vi "Run1Ton.vi"() -> ()   [LabVIEW 2014]
doc: "Use this template to build a producer/consumer design pattern with events to produce queue items. Use this design pattern instead of the User Interface Event Handler pattern for user interfaces when you want to execute code asynchronously in response to an event without slowing the user interface responsiveness."
uses:
  <vilib>/addons/h5labview2/base/hid_t.ctl
  DatasetNames.ctl
  Program Files (x86)/CAEN/Comm/labview/CAENComm.lvlib
panel:
  in  "Delay":u32=1
  out "# elements in queue":i32
  out "Acquiring?":bool
  out "Wfm Plot 2":dbl[][](graph)
  out "# bad reads":i32
  out "Wfm Plot":dbl[][](graph)
  out "Scaler Data":u32[](array[numeric])
  out "Acquisition\nErrors":errorcluster
  in  "Clear Acquisition Errors":bool
  in  "QDC threshold":u16=1
  in  "Start Acquisition":bool
  out "# Events Written":i32
  in  "# Events to\nRecord":i32
  out "Analysis\nErrors":errorcluster
  in  "Calibrate Verniers":bool
  in  "Stop Acquisition":bool
  in  "Configure Output":bool
  in  "Calibrate Pedestals":bool
  in  "stop":bool
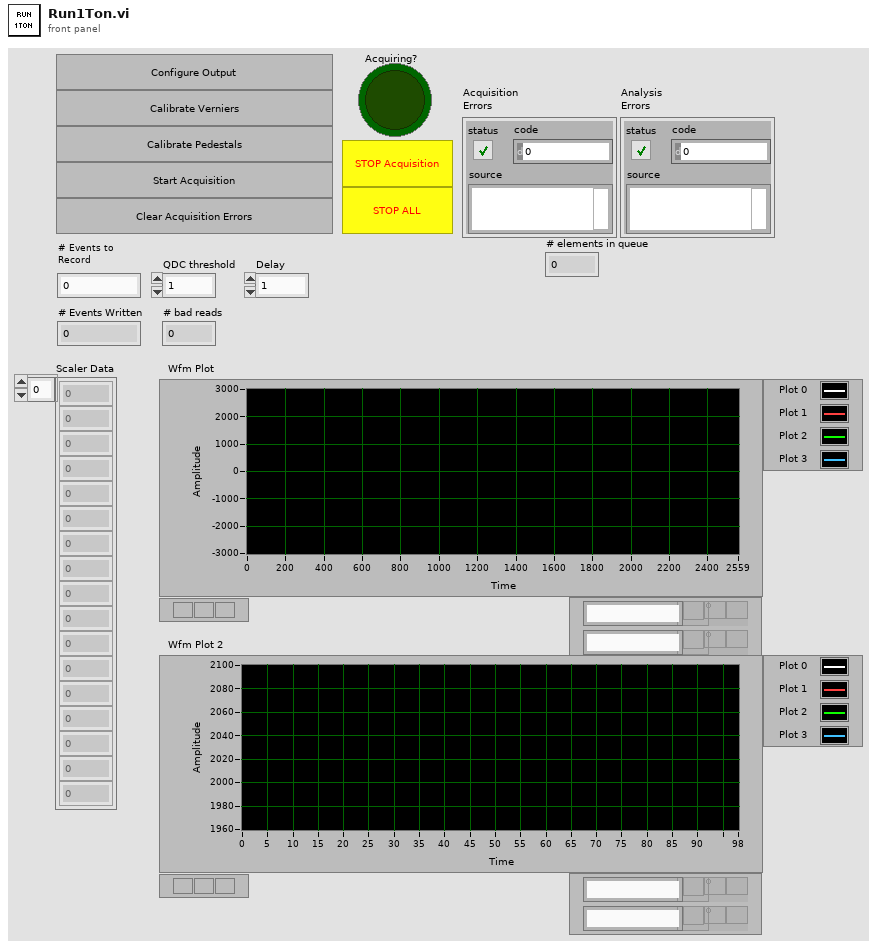
[diagram p1: front panel]
types:
  T1 = typedef "hid_t.ctl" = i32
  T2 = cluster{"State":enum16{"Startup", "Initialise", "Event OK", "Discard Event", "Exit", "Close"}, "Data":variant}
  T3 = typedef "DatasetNames.ctl" = enum16{"TDC", "Scaler", "QDC_1", "QDC_2", "Digitizer_1", "Digitizer_2"}
  T4 = cluster{"TDC Data":u32[], "Scaler Data":u32[], "QDC 1 Data":u32[], "QDC 2 Data":u32[], "Digitizer 1 TRIG_REC":u32, "Digitizer 1 Waveforms":u32[], "Digitizer 2 TRIG_REC":u32, "Digitizer 2 Waveforms":u32[]}
  T5 = enum16{"Startup", "Initialise", "Event OK", "Discard Event", "Exit", "Close"}
  T6 = enum16{"Configure", "Initialise", "Run", "Close"}
  T7 = cluster{"TDC":u32, "Scaler":u32, "QDC 1":u32, "QDC 2":u32, "Digitizer 1":u32, "Digitizer 2":u32}
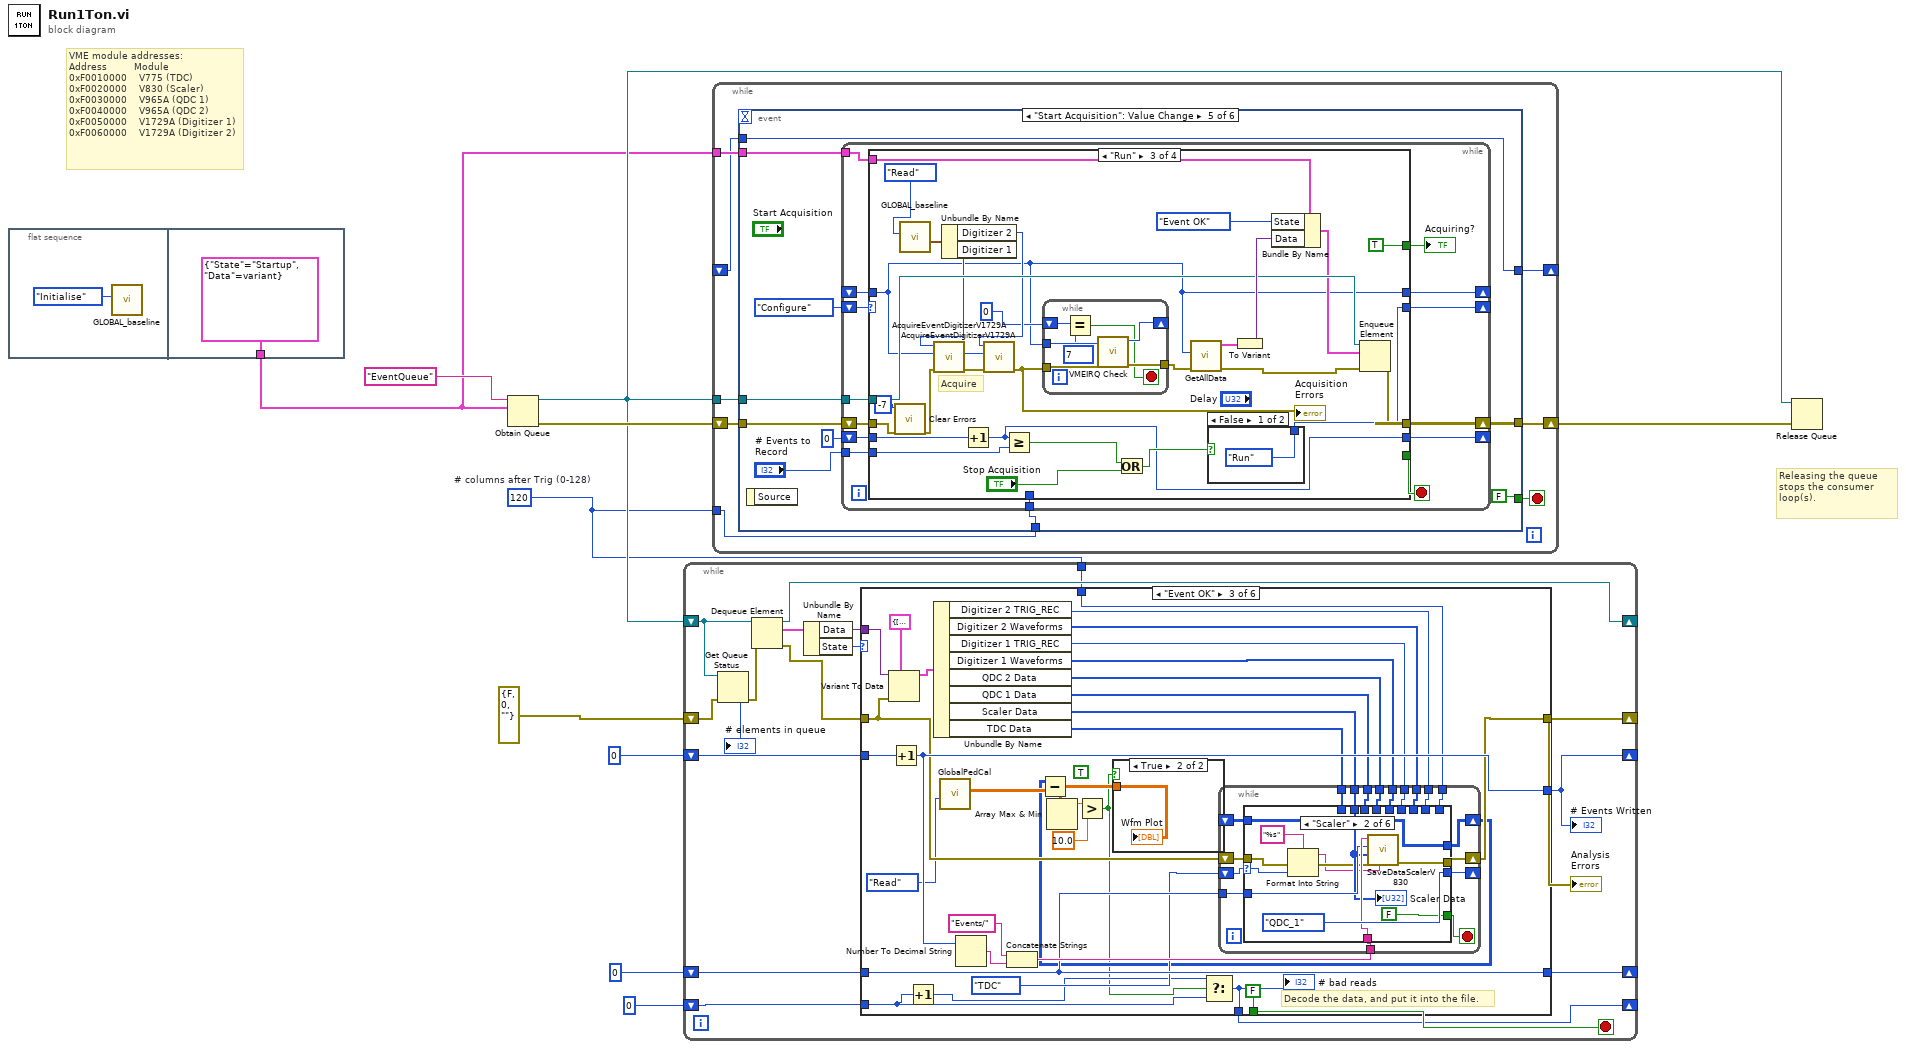
[diagram p0: block diagram]
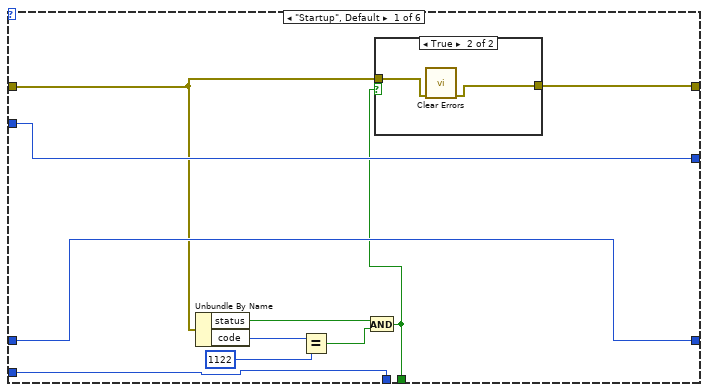
[diagram p2: hidden frame]
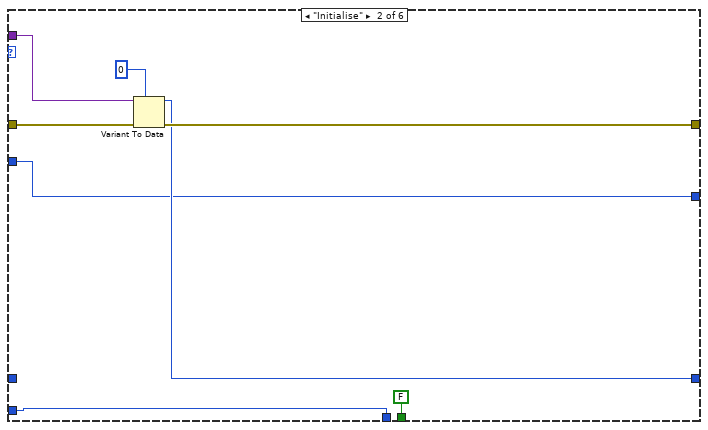
[diagram p4: hidden frame]
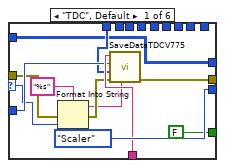
[diagram p6: hidden frame]
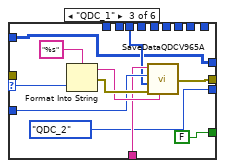
[diagram p7: hidden frame]
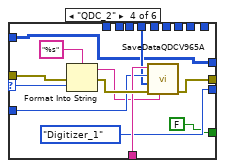
[diagram p8: hidden frame]
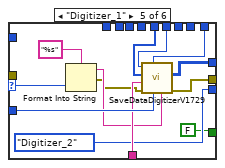
[diagram p9: hidden frame]
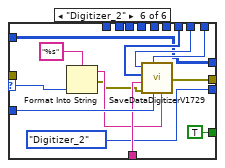
[diagram p10: hidden frame]
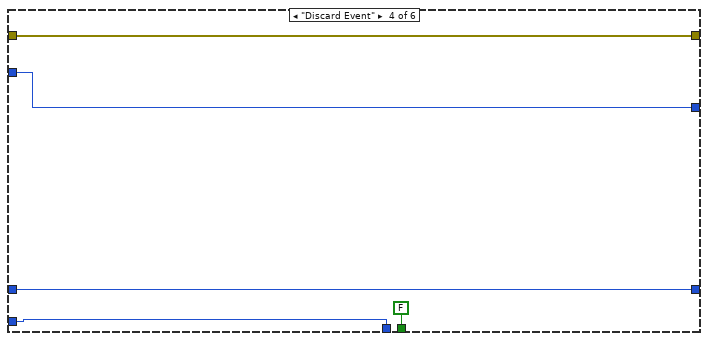
[diagram p11: hidden frame]
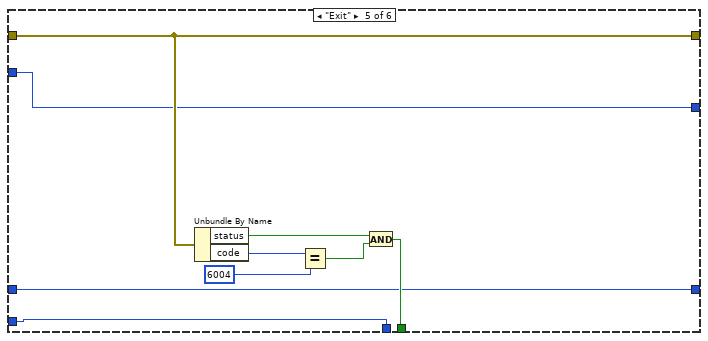
[diagram p12: hidden frame]
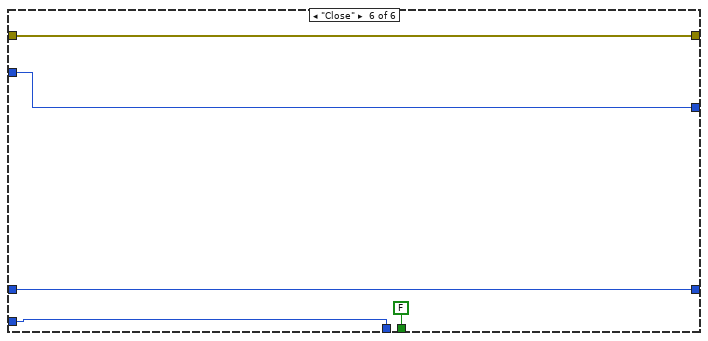
[diagram p13: hidden frame]
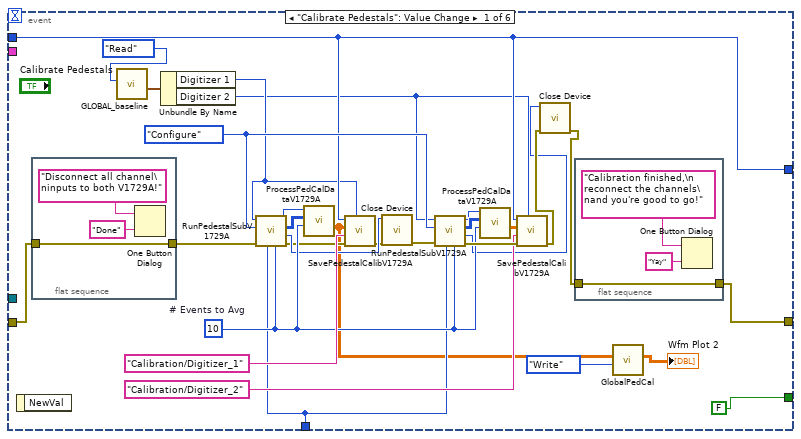
[diagram p14: hidden frame]
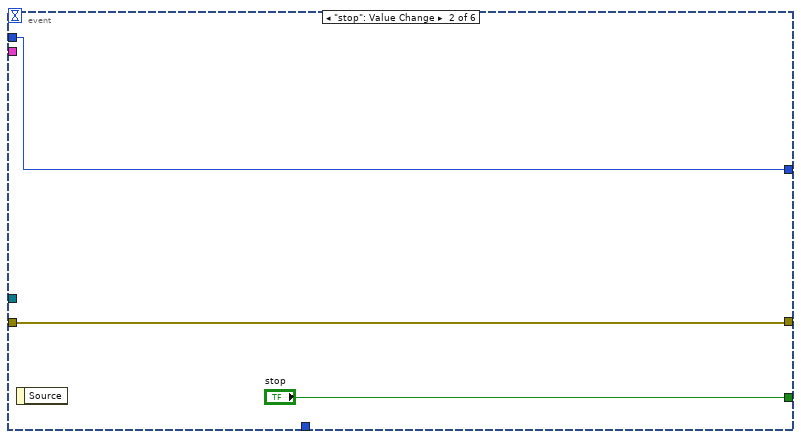
[diagram p15: hidden frame]
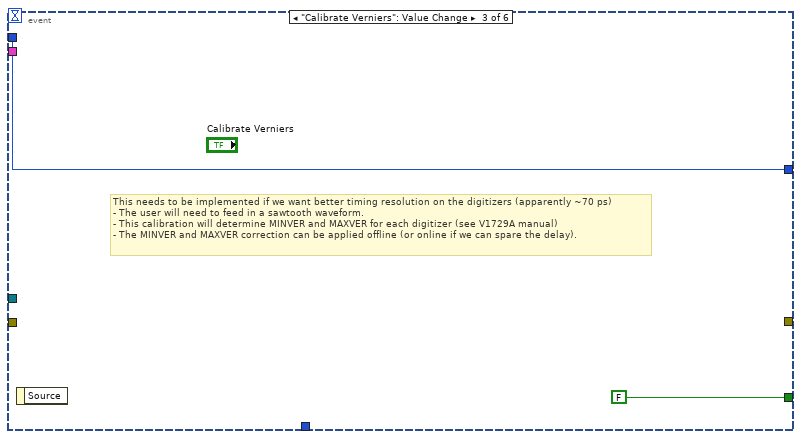
[diagram p16: hidden frame]
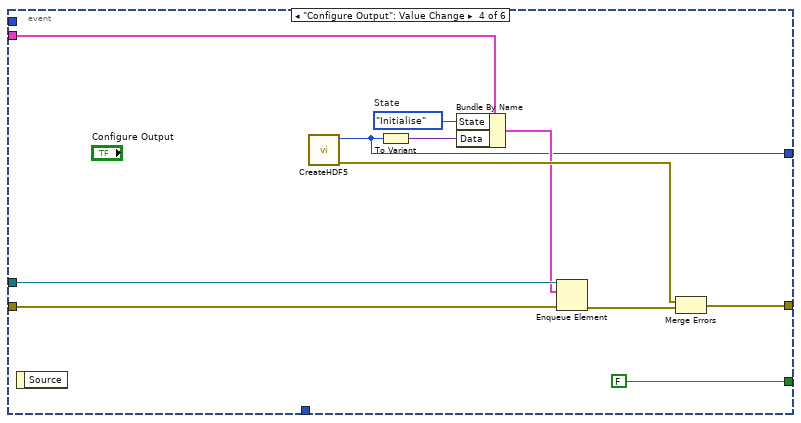
[diagram p17: hidden frame]
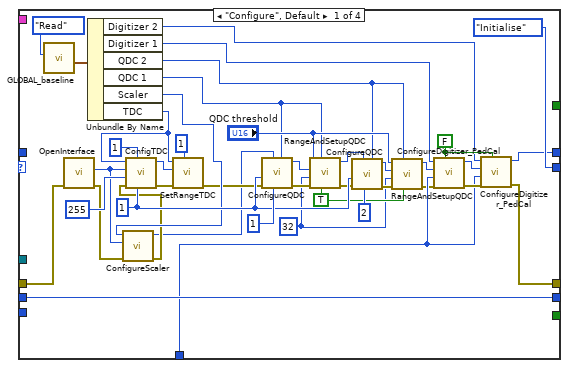
[diagram p18: hidden frame]
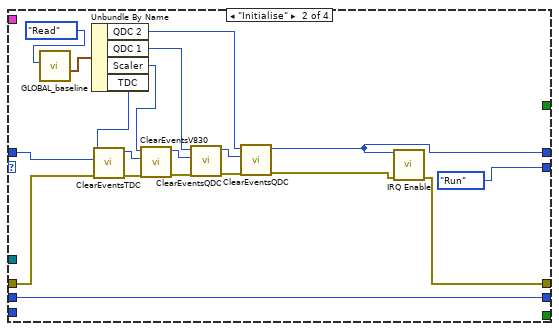
[diagram p19: hidden frame]
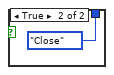
[diagram p20: hidden frame]
diagram:
  w1 = u16 120  # # columns after Trig (0-128)
  # "VME module addresses:\nAddress         Module\n0xF0010000    V775 (TDC)\n0xF0020000    V830 (Scaler)\n0xF0030000    V965A (QDC 1)\n0xF0040000    V965A (QDC 2)\n0xF0050000    V1729A (Digitizer 1)\n0xF0060000    V1729A (Digitizer 2)"
  # "Releasing the queue stops the consumer loop(s)."
  n1 = flat-sequence {
    tunnel: [T2 {"State"=enum."Startup", "Data"=variant}] -> w3
    frame #0 {
      n2 = call "GLOBAL_baseline.vi"("State"=enum16{"Initialise", "Write", "Read"}."Initialise") -> ()  [unwired: 10 in, 1 out]
    }
    frame #1 {
    }
  }
  n3 = Obtain Queue(name (unnamed)="EventQueue", element data type=w3) -> (queue out=w5:refnum<queue>, error out=w10:errorcluster)  [unwired: 3 in, 1 out]
  n4 = while {
    shift-right: [w20] -> _
    shift-left: errorcluster {"status"=FALSE, "code"=0, "source"=""} ("error out") -> [w16]
    shift-right: [w26] -> _
    shift-left: w5 -> [w14]
    shift-right: [w24] -> _
    shift-left: T1 0 ("File Handle") -> [w23]
    tunnel: w1 -> [w22]
    shift-right: [w19] -> _
    shift-left: 0 -> [w21]
    shift-right: [w17] -> _
    shift-left: 0 -> [w18]
    stop <- w25 stop-if-true
    n5 = Get Queue Status(queue=w14, error in (no error)=w16) -> (error out=w15:errorcluster, # elements in queue=→"# elements in queue":i32)  [unwired: 1 in, 6 out]
    n6 = Dequeue Element(queue=w14, error in (no error)=w15) -> (queue out=w26:refnum<queue>, element=w30:T2, error out=w27:errorcluster)  [unwired: 1 in, 1 out]
    n7 = Unbundle By Name(w30) -> ("Data"=w28:variant, "State"=w29:T5)
    n8 = case shown="\"Event OK\"" w29 {
      tunnel: w28 -> [_ w49 w82 _ _ _]
      tunnel: w27 -> [w34 w48 w67 w180 w184 w194]
      tunnel: [w32 w47 w65 w180 w184 w194] -> w20
      tunnel: [w33 FALSE FALSE FALSE w185 FALSE] -> w25
      tunnel: [w36 w46 w71 w178 w183 w192] -> w24
      tunnel: w23 -> [w36 _ w71 w178 w183 w192]
      tunnel: w22 -> [_ _ w73 _ _ _]
      tunnel: w21 -> [w35 w45 w81 w177 w182 w191]
      tunnel: [w35 w45 w80 w177 w182 w191] -> w19
      tunnel: w18 -> [w31 w44 w60 w176 w181 w190]
      tunnel: [w31 w44 w58 w176 w181 w190] -> w17
      frame "Startup", Default {
        n9 = Unbundle By Name(w34) -> ("status"=w40:bool, "code"=w38:i32)
        n10 = Equal?(x=w38, y=1122) -> (x = y?=w39:bool)
        n11 = And(x=w40, y=w39) -> (x .and. y?=w33:bool)
        n12 = case shown="True" w33 {
          tunnel: w34 -> [w41 w43]
          tunnel: [w41 w42] -> w32
          frame False {
          }
          frame True {
            n13 = call <vilib>:"Clear Errors.vi"("error in (no error)"=w43) -> ("error out"=w42:errorcluster)  [unwired: 5 in, 1 out]
          }
        }
      }
      frame "Initialise" {
        n14 = Variant To Data(error in=w48, type=T1 0 ("File Handle"), Variant=w49) -> (data=w46:T1, error out=w47:errorcluster)
      }
      frame "Event OK" {
        (unwired) TRUE
        # "Decode the data, and put it into the file."
        n15 = Variant To Data(error in=w67, type=T4 {"TDC Data"=[], "Scaler Data"=[], "QDC 1 Data"=[], "QDC 2 Data"=[], "Digitizer 1 TRIG_REC"=0, "Digitizer 1 Waveforms"=[], "Digitizer 2 TRIG_REC"=0, "Digitizer 2 Waveforms"=[]}, Variant=w82) -> (data=w76:T4)  [unwired: 1 out]
        n16 = Increment(x=w81) -> (x+1=w80:i32)
        n17 = Increment(x=w60) -> (x+1=w59:i32)
        n18 = Unbundle By Name(w76) -> ("Digitizer 2 TRIG_REC"=w75:u32, "Digitizer 2 Waveforms"=w74:u32[], "Digitizer 1 TRIG_REC"=w56:u32, "Digitizer 1 Waveforms"=w57:u32[], "QDC 2 Data"=w70:u32[], "QDC 1 Data"=w69:u32[], "Scaler Data"=w68:u32[], "TDC Data"=w66:u32[])
        n19 = call "GlobalPedCal.vi"("State"=enum16{"Initialise", "Write", "Read"}."Read") -> ("Data Out"=w55:dbl[][])  [unwired: 10 in]
        n20 = Number To Decimal String(number=w80) -> (decimal integer string=w78:string)  [unwired: 1 in]
        n21 = Concatenate Strings("Events/", w78) -> (w72:string)
        n22 = while {
          tunnel: w75 -> [w102]
          tunnel: w74 -> [w101]
          tunnel: w73 -> [w100]
          tunnel: w72 -> [w99]
          tunnel: w71 -> [w98]
          tunnel: w56 -> [w97]
          tunnel: w57 -> [w96]
          tunnel: w70 -> [w94]
          tunnel: w69 -> [w93]
          shift-right: [w89] -> w65
          shift-left: w67 -> [w95]
          tunnel: w68 -> [w91]
          tunnel: w66 -> [w90]
          shift-right: [w87] -> _
          shift-left: DatasetNames."TDC" -> [w88]
          shift-right: [w86] -> w54
          shift-left: _ -> [w85]
          stop <- w92 stop-if-true
          n23 = case shown="\"Scaler\"" w88 {
            selector: w88 -> [w104 w119 w134 w148 w158 w168]
            tunnel: [w112 w124 w131 w141 w162 w175] -> w89
            tunnel: w102 -> [_ _ _ _ _ w174]
            tunnel: w101 -> [_ _ _ _ _ w173]
            tunnel: w98 -> [w110 w122 w133 w144 w161 w172]
            tunnel: w100 -> [_ _ _ _ w160 w171]
            tunnel: w99 -> [w111 w123 w132 w145 w159 w170]
            tunnel: w97 -> [_ _ _ _ w154 _]
            tunnel: w96 -> [_ _ _ _ w153 _]
            tunnel: w95 -> [w107 w118 _ w147 _ _]
            tunnel: w94 -> [_ _ _ w143 _ _]
            tunnel: w93 -> [_ _ w130 _ _ _]
            tunnel: [DatasetNames."Scaler" DatasetNames."QDC_1" DatasetNames."QDC_2" DatasetNames."Digitizer_1" DatasetNames."Digitizer_2" DatasetNames."Digitizer_2"] -> w87
            tunnel: [FALSE FALSE FALSE FALSE FALSE TRUE] -> w92
            tunnel: w91 -> [_ w121 _ _ _ _]
            tunnel: w90 -> [w109 _ _ _ _ _]
            tunnel: [w103 w115 w127 w138 w150 w163] -> w86
            tunnel: w85 -> [w103 w115 w127 w138 _ w163]
            frame "TDC", Default {
              n24 = Format Into String(format string="%s", error in=w107, w104) -> (resulting string=w105:string, error out=w106:errorcluster)  [unwired: 1 in]
              n25 = call "SaveDataTDCV775.vi"("Module"=w105, "error in (no error)"=w106, "Buff"=w109, "File Handle"=w110, "String"=w111) -> ("error out"=w112:errorcluster)  [unwired: 5 in, 1 out]
            }
            frame "Scaler" {
              n26 = Format Into String(format string="%s", error in=w118, w119) -> (resulting string=w116:string, error out=w117:errorcluster)  [unwired: 1 in]
              n27 = call "SaveDataScalerV830.vi"("Module"=w116, "error in (no error)"=w117, "Buff"=w121, "File Handle"=w122, "Group Name"=w123) -> ("error out"=w124:errorcluster)  [unwired: 6 in]
              "Scaler Data" <- w121
            }
            frame "QDC_1" {
              n28 = Format Into String(format string="%s", w134) -> (resulting string=w135:string, error out=w136:errorcluster)  [unwired: 2 in]
              n29 = call "SaveDataQDCV965A.vi"("Module"=w135, "error in (no error)"=w136, "Buff"=w130, "File Handle"=w133, "String"=w132) -> ("error out"=w131:errorcluster)  [unwired: 5 in, 1 out]
            }
            frame "QDC_2" {
              n30 = Format Into String(format string="%s", error in=w147, w148) -> (resulting string=w142:string, error out=w146:errorcluster)  [unwired: 1 in]
              n31 = call "SaveDataQDCV965A.vi"("Module"=w142, "error in (no error)"=w146, "Buff"=w143, "File Handle"=w144, "String"=w145) -> ("error out"=w141:errorcluster)  [unwired: 5 in, 1 out]
            }
            frame "Digitizer_1" {
              n32 = Format Into String(format string="%s", w158) -> (resulting string=w156:string, error out=w155:errorcluster)  [unwired: 2 in]
              n33 = call "SaveDataDigitizerV1729.vi"("Module"=w156, "File Handle"=w161, "# Samples after Trig"=w160, "error in (no error)"=w155, "String"=w159, "Digitizer Waveforms"=w153, "Digitizer TRIG_REC"=w154) -> ("error out"=w162:errorcluster, "Channel Data"=w150:u16[][])  [unwired: 2 in, 1 out]
            }
            frame "Digitizer_2" {
              n34 = Format Into String(format string="%s", w168) -> (resulting string=w167:string, error out=w166:errorcluster)  [unwired: 2 in]
              n35 = call "SaveDataDigitizerV1729.vi"("Module"=w167, "File Handle"=w172, "# Samples after Trig"=w171, "error in (no error)"=w166, "String"=w170, "Digitizer Waveforms"=w173, "Digitizer TRIG_REC"=w174) -> ("error out"=w175:errorcluster)  [unwired: 2 in, 2 out]
            }
          }
        }
        n36 = Subtract(x=w54, y=w55) -> (x-y=w53:dbl[][])
        n37 = Array Max & Min(array=w53) -> (max value=w62:dbl)  [unwired: 3 out]
        n38 = Greater?(x=w62, y=10.0) -> (0:w52:bool)
        n39 = case shown="True" w52 {
          tunnel: w53 -> [_ w84]
          frame False {
          }
          frame True {
            "Wfm Plot" <- w84
          }
        }
        n40 = Select(t=w59, s=w52, f=w60) -> (s? t:f=w58:i32)
        "# bad reads" <- w58
      }
      frame "Discard Event" {
      }
      frame "Exit" {
        n41 = Unbundle By Name(w184) -> ("status"=w189:bool, "code"=w187:i32)
        n42 = Equal?(x=w187, y=6004) -> (x = y?=w188:bool)
        n43 = And(x=w189, y=w188) -> (x .and. y?=w185:bool)
      }
      frame "Close" {
      }
    }
    "Analysis\nErrors" <- w20
    "# Events Written" <- w19
  }
  n44 = while {
    shift-right: [w200] -> w7
    shift-left: w10 -> [w201]
    tunnel: w5 -> [w202]
    tunnel: w3 -> [w198]
    tunnel: w1 -> [w197]
    shift-right: [w196] -> _
    shift-left: _ -> [w195]
    stop <- w199 stop-if-true
    n45 = event shown="[4] \"Start Acquisition\": Value Change" {
      selector: _ -> [_ _ _ _ _ _]
      dyn-events: _ -> [_ _ _ _ _ _]
      timeout: _ -> [_ _ _ _ _ _]
      tunnel: w202 -> [_ _ _ w246 w259 _]
      tunnel: w201 -> [w207 w240 _ w247 w261 w389]
      tunnel: [w227 w240 _ w250 _ w388] -> w200
      tunnel: [FALSE ("stop") "stop" FALSE ("stop") FALSE ("stop") FALSE ("stop") _] -> w199
      tunnel: w198 -> [_ _ _ w251 w260 _]
      tunnel: w197 -> [w220 _ _ _ w256 _]
      tunnel: [w226 w239 w242 w244 w255 _] -> w196
      tunnel: w195 -> [w226 w239 w242 _ w255 _]
      event "Calibrate Pedestals": Value Change {
        w230 = T6."Configure"
        w221 = 10  # # Events to Avg
        n46 = event-data() -> ()  [unwired: 1 in, 1 out]
        n47 = flat-sequence {
          tunnel: w207 -> [w238]
          tunnel: [w238] -> w217
          frame #0 {
            n48 = One Button Dialog(message="Disconnect all channel\ninputs to both V1729A!", button name ("OK")="Done") -> ()  [unwired: 1 out]
          }
        }
        n49 = call "GLOBAL_baseline.vi"("State"=enum16{"Initialise", "Write", "Read"}."Read") -> ("Addresses Out"=w224:T7)  [unwired: 10 in]
        n50 = Unbundle By Name(w224) -> ("Digitizer 1"=w216:u32, "Digitizer 2"=w213:u32)
        n51 = call "RunPedestalSubV1729A.vi"("# Events to Avg"=w221, "# Samples after Trig"=w220, "error in (no error)"=w217, "Init State"=w230, "VME Base Address in"=w216) -> ("error out"=w210:errorcluster, "handle out"=w215:i32, "Data Out"=w231:u32[][], "Offset"=w209:i16)  [unwired: 3 in]
        n52 = call "ProcessPedCalDataV1729A.vi"("# Events to Avg"=w221, "Data In"=w231, "Offset"=w209) -> ("Channel Data"=w204:dbl[][])  [unwired: 8 in]
        n53 = call "SavePedestalCalibV1729A.vi"("Address"=w216, "error in (no error)"=w210, "Group Name"="Calibration/Digitizer_1", "Data In"=w204, "File Handle"=w226) -> ("error out"=w212:errorcluster)  [unwired: 6 in]
        n54 = call "Close Device.vi"("error in (no error)"=w212, "handle"=w215) -> ("error out"=w211:errorcluster)  [unwired: 9 in]
        n55 = call "RunPedestalSubV1729A.vi"("# Events to Avg"=w221, "# Samples after Trig"=w220, "error in (no error)"=w211, "Init State"=w230, "VME Base Address in"=w213) -> ("error out"=w228:errorcluster, "handle out"=w214:i32, "Data Out"=w229:u32[][], "Offset"=w208:i16)  [unwired: 3 in]
        n56 = call "ProcessPedCalDataV1729A.vi"("# Events to Avg"=w221, "Data In"=w229, "Offset"=w208) -> ("Channel Data"=w205:dbl[][])  [unwired: 8 in]
        n57 = call "SavePedestalCalibV1729A.vi"("Address"=w213, "error in (no error)"=w228, "Group Name"="Calibration/Digitizer_2", "Data In"=w205, "File Handle"=w226) -> ("error out"=w219:errorcluster)  [unwired: 6 in]
        n58 = call "Close Device.vi"("error in (no error)"=w219, "handle"=w214) -> ("error out"=w218:errorcluster)  [unwired: 9 in]
        n59 = flat-sequence {
          tunnel: w218 -> [w233]
          tunnel: [w233] -> w227
          frame #0 {
            n60 = One Button Dialog(message="Calibration finished,\n reconnect the channels\nand you're good to go!", button name ("OK")="Yay") -> ()  [unwired: 1 out]
          }
        }
        n61 = call "GlobalPedCal.vi"("State"=enum16{"Initialise", "Write", "Read"}."Write", "Data In"=w204) -> ("Data Out"=→"Wfm Plot 2":dbl[][])  [unwired: 9 in]
      }
      event "stop": Value Change {
        n62 = event-data() -> ()  [unwired: 1 in, 1 out]
      }
      event "Calibrate Verniers": Value Change {
        # "This needs to be implemented if we want better timing resolution on the digitizers (apparently ~70 ps)\n- The user will need to feed in a sawtooth waveform.\n- This calibration will determine MINVER and MAXVER for each digitizer (see V1729A manual)\n- The MINVER and MAXVER correction can be applied offline (or online if we can spare the delay)."
        n63 = event-data() -> ()  [unwired: 1 in, 1 out]
      }
      event "Configure Output": Value Change {
        w252 = T5."Initialise"  # State
        n64 = event-data() -> ()  [unwired: 1 in, 1 out]
        n65 = call "CreateHDF5.vi"() -> ("error out"=w249:errorcluster, "File Handle"=w244:T1)  [unwired: 10 in]
        n66 = To Variant(anything=w244) -> (Variant=w253:variant)
        n67 = Bundle By Name(cluster=w251, "State"=w252, "Data"=w253) -> (w245:T2)
        n68 = Enqueue Element(queue=w246, element=w245, error in (no error)=w247) -> (error out=w248:errorcluster)  [unwired: 1 in, 2 out]
        n69 = Merge Errors(w249, w248) -> (w250:errorcluster)
      }
      event "Start Acquisition": Value Change {
        n70 = event-data() -> ()  [unwired: 1 in, 1 out]
        n71 = while {
          shift-right: [w272] -> _
          shift-left: T6."Configure" -> [w277]
          shift-right: [w275] -> _
          shift-left: w261 -> [w276]
          shift-right: [w274] -> _
          shift-left: _ -> [w273]
          tunnel: w260 -> [w271]
          tunnel: w259 -> [w270]
          tunnel: "# Events to\nRecord" -> [w268]
          shift-right: [w266] -> _
          shift-left: 0 -> [w269]
          tunnel: w256 -> [w265]
          stop <- w267 stop-if-true
          n72 = case shown="\"Run\"" w277 {
            tunnel: w276 -> [w318 w334 w366 w378]
            tunnel: [w303 w335 w360 w384] -> w275
            tunnel: [w302 w325 w340 w376] -> w274
            tunnel: w273 -> [_ w333 w340 w376]
            tunnel: [T6."Initialise" T6."Run" w357 T6."Close"] -> w272
            tunnel: w271 -> [_ _ w363 w380]
            tunnel: w270 -> [_ _ w362 w383]
            tunnel: w269 -> [w316 w336 w356 w385]
            tunnel: w268 -> [_ _ w355 _]
            tunnel: [_ _ _ TRUE] -> w267
            tunnel: [w316 w336 w353 w385] -> w266
            tunnel: w265 -> [w305 _ _ _]
            tunnel: [_ _ TRUE _] -> w264
            frame "Configure", Default {
              w294 = u16 32 ("High range threshold")
              w295 = TRUE ("Count only accepted trigs?\n(else all trigs)")
              w309 = u16 1 ("# Evts to Acquire")
              w304 = FALSE ("Software Trig?")
              n73 = call "GLOBAL_baseline.vi"("State"=enum16{"Initialise", "Write", "Read"}."Read") -> ("Addresses Out"=w289:T7)  [unwired: 10 in]
              n74 = call "OpenInterface.vi"("error in (no error)"=w318) -> ("error out"=w283:errorcluster, "handle"=w282:i32)  [unwired: 8 in, 1 out]
              n75 = Unbundle By Name(w289) -> ("Digitizer 2"=w284:u32, "Digitizer 1"=w285:u32, "QDC 2"=w286:u32, "QDC 1"=w287:u32, "Scaler"=w281:u32, "TDC"=w288:u32)
              n76 = call "ConfigureScaler.vi"("error in (no error)"=w283, "handle"=w282, "VME Base Address"=w281) -> ("error out"=w280:errorcluster, "handle out"=w278:i32)  [unwired: 6 in, 1 out]
              n77 = call "ConfigTDC.vi"("# Evts to Acquire"=w309, "Interrupt Level"=u16 1, "error in (no error)"=w280, "FSR setting"=u16 255, "handle"=w282, "VME Base Address"=w288) -> ("error out"=w313:errorcluster, "handle out"=w312:i32)  [unwired: 4 in]
              n78 = call "SetRangeTDC.vi"("Low Range threshold"=u16 1, "error in (no error)"=w313, "handle"=w312, "VME module Base Address"=w288) -> ("error out"=w279:errorcluster)  [unwired: 5 in, 2 out]
              n79 = call "ConfigureQDC.vi"("VME module Base Address"=w287, "IRQ Lvl"=u16 1, "handle"=w278, "error in (no error)"=w279, "# of events before transfer (max 32)"=w309) -> ("error out"=w301:errorcluster, "handle out"=w300:i32)  [unwired: 5 in]
              n80 = call "RangeAndSetupQDC.vi"("Count only accepted trigs?\n(else all trigs)"=w295, "VME module Base Address"=w287, "error in (no error)"=w301, "High range threshold"=w294, "handle in"=w300, "Low Range threshold"="QDC threshold") -> ("error out"=w299:errorcluster, "handle out"=w298:i32)  [unwired: 4 in]
              n81 = call "ConfigureQDC.vi"("VME module Base Address"=w286, "IRQ Lvl"=u16 2, "handle"=w298, "error in (no error)"=w299, "# of events before transfer (max 32)"=w309) -> ("error out"=w297:errorcluster, "handle out"=w292:i32)  [unwired: 5 in]
              n82 = call "RangeAndSetupQDC.vi"("Count only accepted trigs?\n(else all trigs)"=w295, "VME module Base Address"=w286, "error in (no error)"=w297, "High range threshold"=w294, "handle in"=w292, "Low Range threshold"="QDC threshold") -> ("error out"=w296:errorcluster, "handle out"=w291:i32)  [unwired: 4 in]
              n83 = call "ConfigureDigitizer_PedCal.vi"("Software Trig?"=w304, "error in (no error)"=w296, "# Samples after Trig"=w305, "handle"=w291, "VME Base Address"=w285) -> ("error out"=w307:errorcluster, "handle out"=w306:i32)  [unwired: 4 in, 1 out]
              n84 = call "ConfigureDigitizer_PedCal.vi"("Software Trig?"=w304, "error in (no error)"=w307, "# Samples after Trig"=w305, "handle"=w306, "VME Base Address"=w284) -> ("error out"=w303:errorcluster, "handle out"=w302:i32)  [unwired: 4 in, 1 out]
            }
            frame "Initialise" {
              n85 = call "GLOBAL_baseline.vi"("State"=enum16{"Initialise", "Write", "Read"}."Read") -> ("Addresses Out"=w323:T7)  [unwired: 10 in]
              n86 = Unbundle By Name(w323) -> ("QDC 2"=w319:u32, "QDC 1"=w320:u32, "Scaler"=w321:u32, "TDC"=w322:u32)
              n87 = call "ClearEventsTDC.vi"("error in (no error)"=w334, "handle"=w333, "VME module Base Address"=w322) -> ("error out"=w332:errorcluster, "handle out"=w331:i32)  [unwired: 6 in, 1 out]
              n88 = call "ClearEventsV830.vi"("error in (no error)"=w332, "handle in"=w331, "VME Base Address"=w321) -> ("error out"=w330:errorcluster, "handle out"=w329:i32)  [unwired: 7 in]
              n89 = call "ClearEventsQDC.vi"("error in (no error)"=w330, "handle"=w329, "VME module Base Address"=w320) -> ("error out"=w328:errorcluster, "handle out"=w327:i32)  [unwired: 6 in, 1 out]
              n90 = call "ClearEventsQDC.vi"("error in (no error)"=w328, "handle"=w327, "VME module Base Address"=w319) -> ("error out"=w326:errorcluster, "handle out"=w325:i32)  [unwired: 6 in, 1 out]
              n91 = call "IRQ Enable.vi"("error in (no error)"=w326, "handle"=w325) -> ("error out"=w335:errorcluster)  [unwired: 9 in]
            }
            frame "Run" {
              # "Acquire"
              n92 = call <vilib>:"Clear Errors.vi"("error in (no error)"=w366, "specific error code to clear (0: all)"=-7) -> ("error out"=w345:errorcluster)  [unwired: 4 in, 1 out]
              n93 = call "GLOBAL_baseline.vi"("State"=enum16{"Initialise", "Write", "Read"}."Read") -> ("Addresses Out"=w351:T7)  [unwired: 10 in]
              n94 = Unbundle By Name(w351) -> ("Digitizer 2"=w347:u32, "Digitizer 1"=w350:u32)
              n95 = call "AcquireEventDigitizerV1729A.vi"("error in (no error)"=w345, "handle in"=w340, "VME Base Address"=w350) -> ("error out"=w349:errorcluster, "handle out"=w348:i32)  [unwired: 7 in]
              n96 = Increment(x=w356) -> (x+1=w353:i32)
              n97 = call "AcquireEventDigitizerV1729A.vi"("error in (no error)"=w349, "handle in"=w348, "VME Base Address"=w347) -> ("error out"=w346:errorcluster)  [unwired: 7 in, 1 out]
              "Acquisition\nErrors" <- w346
              n98 = Greater Or Equal?(x=w353, y=w355) -> (x >= y?=w354:bool)
              n99 = while {
                tunnel: w346 -> [w373]
                tunnel: [w372] -> w338
                tunnel: w340 -> [w371]
                shift-right: [w370] -> _
                shift-left: u8 0 ("Mask") -> [w368]
                stop <- w367 stop-if-true
                n100 = Equal?(x=w368, y=u8 7) -> (x = y?=w367:bool)
                n101 = call "VMEIRQ Check.vi"("error in (no error)"=w373, "VMEhandle"=w371) -> ("error out"=w372:errorcluster, "Mask"=w370:u8)  [unwired: 8 in]
              }
              n102 = Or(x=w354, y="Stop Acquisition") -> (x .or. y?=w358:bool)
              n103 = call "GetAllData.vi"("error in (no error)"=w338, "handle in"=w340) -> ("error out"=w339:errorcluster, "Data cluster"=w343:T4)  [unwired: 7 in, 1 out]
              n104 = case shown="False" w358 {
                tunnel: [T6."Run" T6."Close"] -> w357
                frame False {
                }
                frame True {
                }
              }
              n105 = To Variant(anything=w343) -> (Variant=w365:variant)
              n106 = Bundle By Name(cluster=w363, "State"=T5."Event OK", "Data"=w365) -> (w361:T2)
              n107 = Enqueue Element(queue=w362, element=w361, error in (no error)=w339) -> (error out=w360:errorcluster)  [unwired: 1 in, 2 out]
            }
            frame "Close" {
              n108 = call "Close Device.vi"("error in (no error)"=w378, "handle"=w376) -> ("error out"=w377:errorcluster)  [unwired: 9 in]
              n109 = Bundle By Name(cluster=w380, "State"=T5."Close", "Data"=variant) -> (w379:T2)
              n110 = Enqueue Element(queue=w383, element=w379, error in (no error)=w377) -> (error out=w384:errorcluster)  [unwired: 1 in, 2 out]
            }
          }
          "Acquiring?" <- w264
        }
      }
      event "Clear Acquisition Errors": Value Change {
        n111 = event-data() -> ()  [unwired: 1 in, 2 out]
        n112 = call <vilib>:"Clear Errors.vi"("error in (no error)"=w389) -> ("error out"=w388:errorcluster)  [unwired: 5 in, 1 out]
      }
    }
  }
  n113 = Release Queue(queue=w5, error in (no error)=w7) -> ()  [unwired: 1 in, 3 out]
